vi "Control Front Panel State.vi"(8 "error out":errorcluster, 9 "Front Panel Window:Behavior":T1(ring)=enum."Default", 10 "Argument":T2="Open", 11 "Core.Current VI Reference":refnum<vi>) -> (0 "error out":errorcluster, 3 "reference out":refnum<vi>)   [LabVIEW 2021]
doc: "control VI Front panel.\n2014-11-14 16:09:09\n蒋松"
uses:
  <userlib>/John_Lib/Control/Panel State.ctl
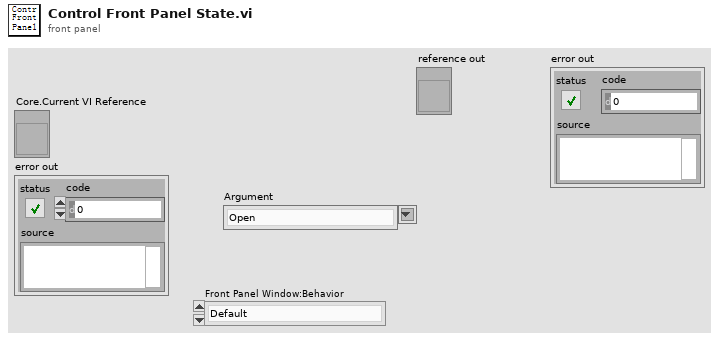
[diagram p1: front panel]
types:
  T1 = enum32{"Invalid", "Default", "Floating", "Floating/Auto-Hide", "Modal"}
  T2 = typedef "Panel State.ctl" = string
  T3 = enum32{"Invalid", "Standard", "Closed", "Hidden", "Minimized", "Maximized"}
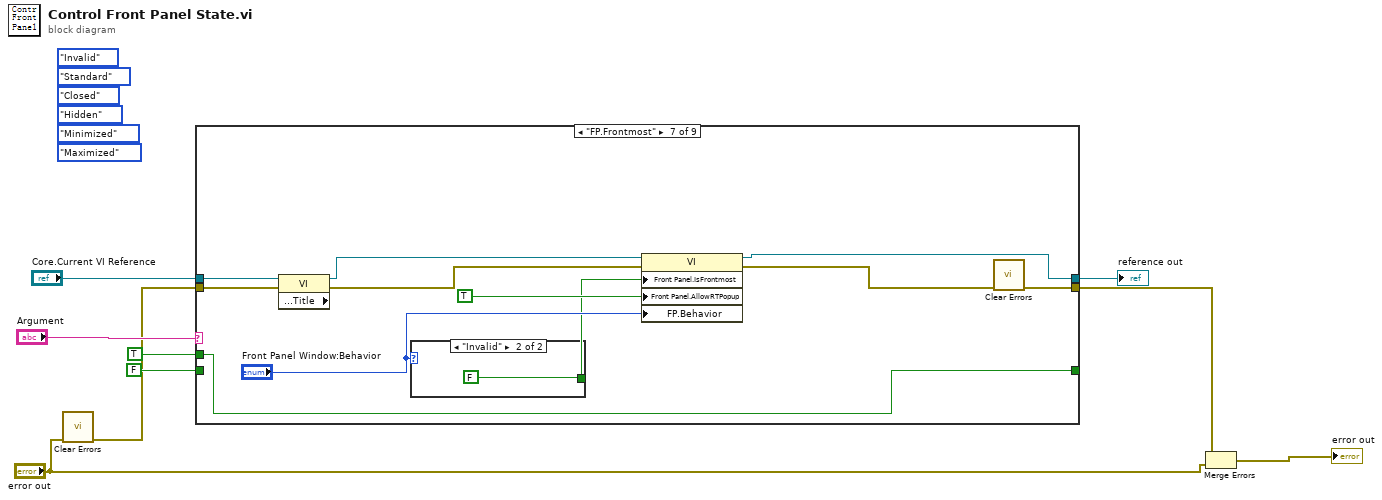
[diagram p0: block diagram]
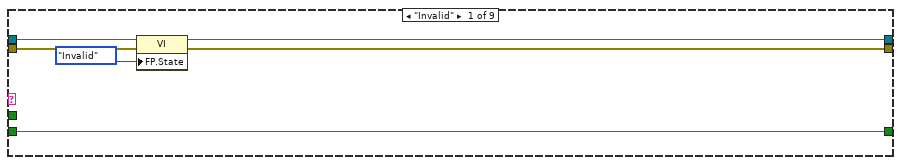
[diagram p2: hidden frame]
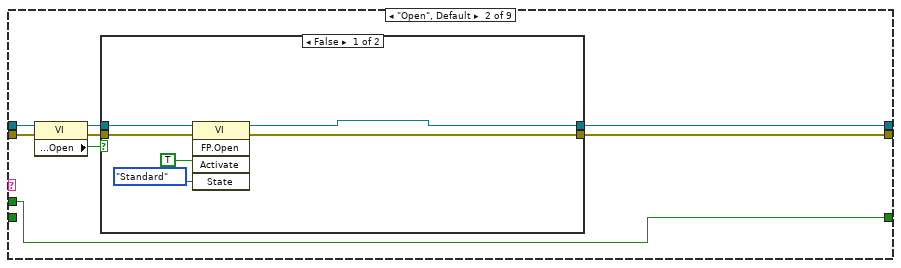
[diagram p3: hidden frame]
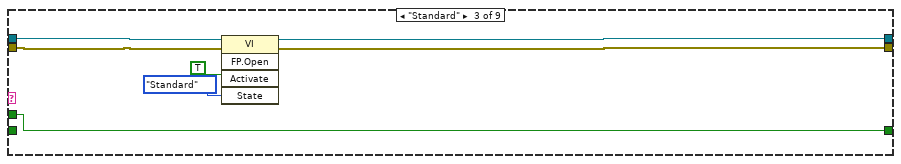
[diagram p5: hidden frame]
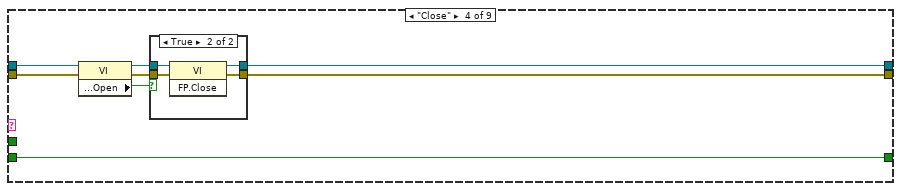
[diagram p6: hidden frame]
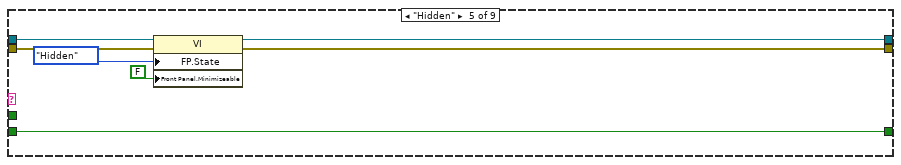
[diagram p8: hidden frame]
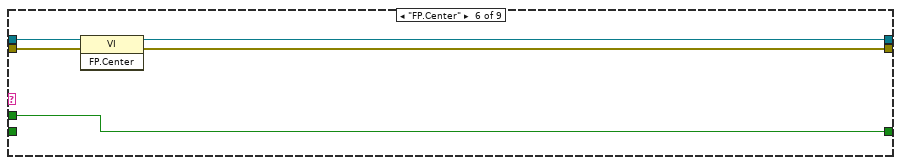
[diagram p9: hidden frame]
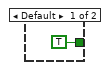
[diagram p10: hidden frame]
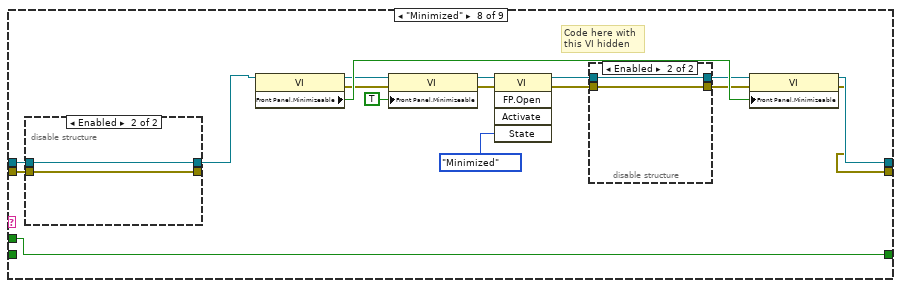
[diagram p11: hidden frame]
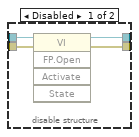
[diagram p12: hidden frame]
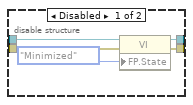
[diagram p13: hidden frame]
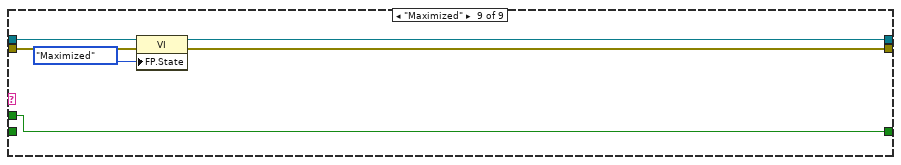
[diagram p14: hidden frame]
diagram:
  (unwired) T3."Maximized" ("State")
  (unwired) T3."Minimized" ("State")
  (unwired) T3."Hidden" ("State")
  (unwired) T3."Closed" ("State")
  (unwired) T3."Standard" ("State")
  (unwired) T3."Invalid" ("State")
  n1 = call <vilib>:"Clear Errors.vi"("error in (no error)"="error out") -> ("error out"=w3:errorcluster)  [unwired: 5 in, 1 out]
  n2 = case shown="\"FP.Frontmost\"" "Argument" {
    tunnel: w3 -> [w13 w21 w37 w45 w59 w63 w74 w93 w111]
    tunnel: [w12 w23 w33 w46 w58 w62 w73 w78 w110] -> w6
    tunnel: "Core.Current VI Reference" -> [w14 w22 w38 w43 w56 w64 w75 w94 w112]
    tunnel: [w11 w17 w34 w40 w53 w61 w70 w79 w109] -> w7
    tunnel: [w10 w16 w32 w39 w54 w60 w72 w92 w108] -> _
    tunnel: FALSE ("Front Panel Window:Minimizable") -> [w10 _ _ w39 w54 _ _ _ _]
    tunnel: TRUE ("Front Panel Window:Minimizable") -> [_ w16 w32 _ _ w60 w72 w92 w108]
    frame "Invalid" {
      n3 = property class="VI"(reference=w14, error in=w13, "FP.State"=T3."Invalid" ("Front Panel Window:State")) -> (reference out=w11:refnum<vi>, error out=w12:errorcluster)
    }
    frame "Open", Default {
      n4 = property class="VI"(reference=w22, error in=w21) -> (reference out=w19:refnum<vi>, error out=w20:errorcluster, "Front Panel.Open"=w18:bool)
      n5 = case shown="False" w18 {
        tunnel: [w24 w31] -> w23
        tunnel: w20 -> [w27 w31]
        tunnel: w19 -> [w26 w30]
        tunnel: [w25 w30] -> w17
        frame False {
          n6 = invoke class="VI" method="FP.Open"(reference=w26, error in=w27, "Activate"=TRUE, "State"=T3."Standard") -> (reference out=w25:refnum<vi>, error out=w24:errorcluster)  [unwired: 1 in, 3 out]
        }
        frame True {
        }
      }
    }
    frame "Standard" {
      n7 = invoke class="VI" method="FP.Open"(reference=w38, error in=w37, "Activate"=TRUE, "State"=T3."Standard") -> (reference out=w34:refnum<vi>, error out=w33:errorcluster)  [unwired: 1 in, 3 out]
    }
    frame "Close" {
      n8 = property class="VI"(reference=w43, error in=w45) -> (reference out=w42:refnum<vi>, error out=w44:errorcluster, "Front Panel.Open"=w41:bool)
      n9 = case shown="True" w41 {
        tunnel: [w48 w52] -> w46
        tunnel: w44 -> [w48 w51]
        tunnel: w42 -> [w47 w50]
        tunnel: [w47 w49] -> w40
        frame False {
        }
        frame True {
          n10 = invoke class="VI" method="FP.Close"(reference=w50, error in=w51) -> (reference out=w49:refnum<vi>, error out=w52:errorcluster)  [unwired: 1 in, 1 out]
        }
      }
    }
    frame "Hidden" {
      n11 = property class="VI"(reference=w56, error in=w59, "FP.State"=T3."Hidden" ("Front Panel Window:State"), "Front Panel.Minimizeable"=FALSE ("Front Panel Window:Minimizable")) -> (reference out=w53:refnum<vi>, error out=w58:errorcluster)
    }
    frame "FP.Center" {
      n12 = invoke class="VI" method="FP.Center"(reference=w64, error in=w63) -> (reference out=w61:refnum<vi>, error out=w62:errorcluster)  [unwired: 1 in, 1 out]
    }
    frame "FP.Frontmost" {
      n13 = property class="VI" props=["Front Panel.Title"](reference=w75, error in=w74) -> (reference out=w71:refnum<vi>, error out=w66:errorcluster)  [unwired: 1 out]
      n14 = case shown="\"Invalid\"" "Front Panel Window:Behavior" {
        tunnel: [TRUE ("Front Panel Window:Is Frontmost") FALSE ("Front Panel Window:Is Frontmost")] -> w67
        frame Default {
        }
        frame "Invalid" {
        }
      }
      n15 = property class="VI"(reference=w71, error in=w66, "Front Panel.IsFrontmost"=w67, "Front Panel.AllowRTPopup"=TRUE ("Front Panel Window:Allow Runtime PopUp"), "FP.Behavior"="Front Panel Window:Behavior") -> (reference out=w70:refnum<vi>, error out=w65:errorcluster)
      n16 = call <vilib>:"Clear Errors.vi"("error in (no error)"=w65) -> ("error out"=w73:errorcluster)  [unwired: 5 in, 1 out]
    }
    frame "Minimized" {
      # "Code here with\nthis VI hidden"
      n17 = disable-structure shown="Enabled" {
        disable-tunnel: w94 -> [w104 w107]
        disable-tunnel: w93 -> [w103 w106]
        disable-tunnel: [w102 w106] -> _
        disable-tunnel: [w101 w107] -> w80
        frame Disabled {
          n18 = property class="VI"(reference=w104, error in=w103, "FP.State"=T3."Minimized" ("Front Panel Window:State")) -> (reference out=w101:refnum<vi>, error out=w102:errorcluster)
        }
        frame Enabled {
        }
      }
      n19 = property class="VI"(reference=w80) -> (reference out=w90:refnum<vi>, error out=w89:errorcluster, "Front Panel.Minimizeable"=w91:bool)  [unwired: 1 in]
      n20 = property class="VI"(reference=w90, error in=w89, "Front Panel.Minimizeable"=TRUE ("Front Panel Window:Minimizable")) -> (reference out=w84:refnum<vi>, error out=w83:errorcluster)
      n21 = invoke class="VI" method="FP.Open"(reference=w84, error in=w83, "State"=T3."Minimized") -> (reference out=w86:refnum<vi>, error out=w85:errorcluster)  [unwired: 2 in, 3 out]
      n22 = disable-structure shown="Enabled" {
        disable-tunnel: [w98 w100] -> w88
        disable-tunnel: [w97 w99] -> w87
        disable-tunnel: w86 -> [w96 w100]
        disable-tunnel: w85 -> [w95 w99]
        frame Disabled {
          n23 = invoke class="VI" method="FP.Open"(reference=w96, error in=w95) -> (reference out=w98:refnum<vi>, error out=w97:errorcluster)  [unwired: 3 in, 3 out]
        }
        frame Enabled {
        }
      }
      n24 = property class="VI"(reference=w88, error in=w87, "Front Panel.Minimizeable"=w91) -> (reference out=w79:refnum<vi>, error out=w78:errorcluster)
    }
    frame "Maximized" {
      n25 = property class="VI"(reference=w112, error in=w111, "FP.State"=T3."Maximized" ("Front Panel Window:State")) -> (reference out=w109:refnum<vi>, error out=w110:errorcluster)
    }
  }
  "reference out" <- w7
  n26 = Merge Errors(w6, "error out") -> (→"error out":errorcluster)
